vi "Configure View Model.vi"(8 "error in (no error)":errorcluster, 10 "Control View Model":refnum<class "Control View Model.lvclass">, 11 "Control View In":refnum<class "Control View.lvclass">) -> (0 "error out":errorcluster, 3 "Control View Out":refnum<class "Control View.lvclass">)   [LabVIEW 2020]
uses:
  Control View.lvclass
  Control View Model/Control View Model.lvclass
  Control View.lvclass/Control View.ctl
  C:/Users/anton/Documents/GitHub/triarc-debugger/source/Debug View/Debug View.lvclass
  C:/Users/anton/Documents/GitHub/triarc-debugger/source/Control View/Control View.lvclass
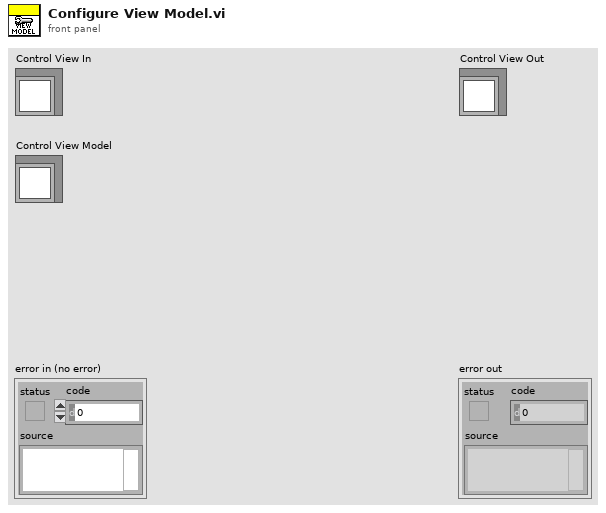
[diagram p1: front panel]
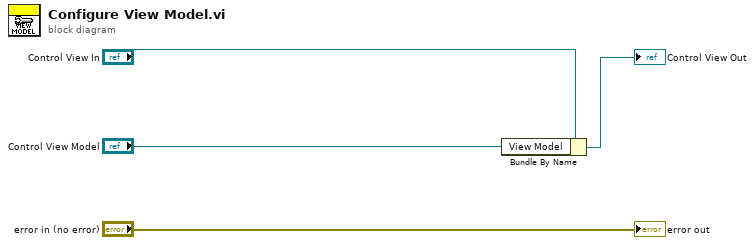
[diagram p0: block diagram]
diagram:
  n1 = Bundle By Name(cluster="Control View In", "View Model"="Control View Model") -> (→"Control View Out":refnum<class "Control View.lvclass">)
  "error out" <- "error in (no error)"
